vi "System Event Formatter (SubVI).vi"(11 "Message Cluster In":T1={"Message Tag"="", "Message Body"="", "Snooze Time (s)"=0.0, "Snooze Alert?"=TRUE, "Log Event?"=TRUE, "Send Email"=0}) -> (3 "Log Message":string)   [LabVIEW 2019]
uses:
  Globals and Definitions/System Message.ctl
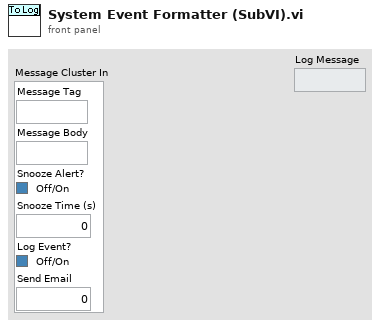
[diagram p1: front panel]
types:
  T1 = typedef "System Message.ctl" = cluster{"Message Tag":string, "Message Body":string, "Snooze Time (s)":dbl, "Snooze Alert?":bool, "Log Event?":bool, "Send Email":i32}
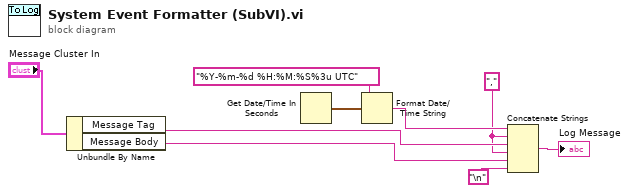
[diagram p0: block diagram]
diagram:
  w3 = ","
  n1 = Unbundle By Name("Message Cluster In") -> ("Message Tag"=w6:string, "Message Body"=w5:string)
  n2 = Get Date/Time In Seconds() -> (seconds since 1Jan1904=w1:timestamp)
  n3 = Format Date/Time String(time format string (%c)="%Y-%m-%d %H:%M:%S%3u UTC", seconds (now)=w1) -> (date/time string=w8:string)  [unwired: 1 in]
  n4 = Concatenate Strings(w8, w3, w6, w3, w5, "\n") -> (→"Log Message":string)
